vi "S7COMM - Timestamp to Siemens Date & Time.vi"(8 "error in":errorcluster, 11 "Time Stamp":timestamp) -> (0 "error out":errorcluster, 1 "DT":T1 {"Weekday" items=["Sunday"=1, "Monday"=2, "Tuesday"=3, "Wednesday"=4, "Thursday"=5, "Friday"=6, "Saturday"=7]; "Month" items=["Jan"=1, "Feb"=2, "Mar"=3, "Apr"=4, "May"=5, "Jun"=6, "Jul"=7, "Aug"=8, "Sep"=9, "Oct"=10, "Nov"=11, "Dec"=12]}, 3 "S7 DATE_AND_TIME":u8[](array[numeric]))   [LabVIEW 2014, in "S7NetCom.lvclass"]
uses:
  S7NetCom.lvclass
  S7COMM - Siemens Date & Time--cluster.ctl
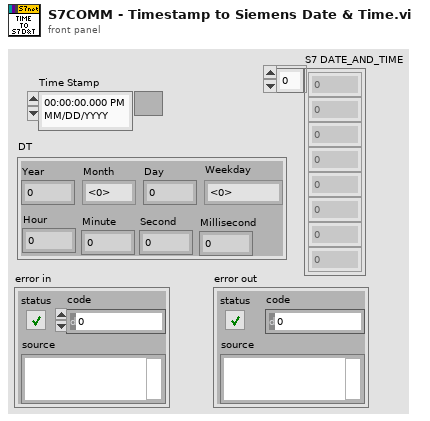
[diagram p1: front panel]
types:
  T1 = typedef "S7NetCom.lvclass/S7COMM - Siemens Date & Time--cluster.ctl" = cluster{"Year":i32, "Month":u8, "Day":u8, "Hour":u8, "Minute":u8, "Second":u8, "Millisecond":u32, "Weekday":u8}
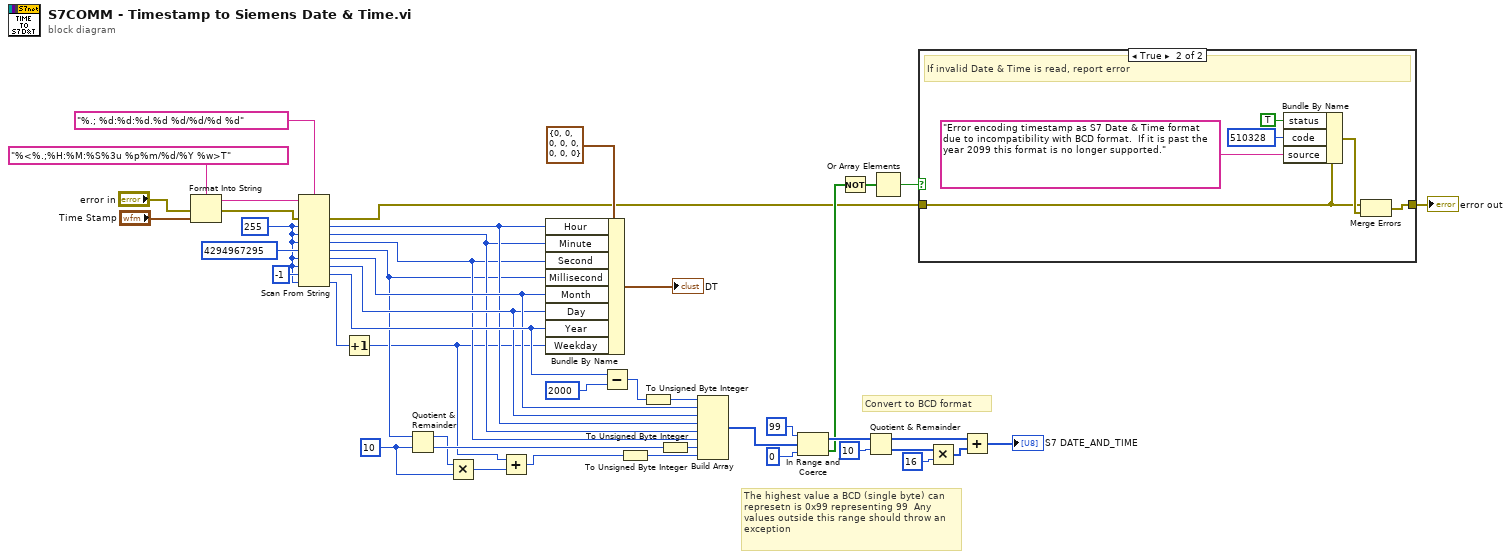
[diagram p0: block diagram]
diagram:
  w22 = u32 10 ("y")
  w36 = u8 255
  # "Convert to BCD format"
  # "The highest value a BCD (single byte) can represetn is 0x99 representing 99  Any values outside this range should throw an exception"
  n1 = Format Into String(format string="%<%.;%H:%M:%S%3u %p%m/%d/%Y %w>T", error in="error in", "Time Stamp") -> (resulting string=w44:string, error out=w39:errorcluster)  [unwired: 1 in]
  n2 = Scan From String(format string="%.; %d:%d:%d.%d %d/%d/%d %d", input string=w44, error in=w39, default 1=w36, default 2=w36, default 3=w36, default 4=u32 4294967295, default 5=w36, default 6=w36, default 7=-1 ("default value 7"), default 8=w36) -> (error out=w3:errorcluster, output 1=w28:u8, output 2=w27:u8, output 3=w26:u8, output 4=w25:u32, output 5=w30:u8, output 6=w29:u8, output 7=w34:i32, output 8=w35:u8)  [unwired: 1 in, 2 out]
  n3 = Increment(x=w35) -> (x+1=w20:u8)
  n4 = Quotient & Remainder(x=w25, y=w22) -> (x-y*floor(x/y)=w23:u32, floor(x/y)=w24:u32)
  n5 = Multiply(x=w23, y=w22) -> (x*y=w21:u32)
  n6 = Add(x=w20, y=w21) -> (x+y=w19:u32)
  n7 = Bundle By Name(cluster=T1 {"Year"=0, "Month"=0, "Day"=0, "Hour"=0, "Minute"=0, "Second"=0, "Millisecond"=0, "Weekday"=0} ("DT"), "Hour"=w28, "Minute"=w27, "Second"=w26, "Millisecond"=w25, "Month"=w30, "Day"=w29, "Year"=w34, "Weekday"=w20) -> (→"DT":T1)
  n8 = Subtract(x=w34, y=2000) -> (x-y=w32:i32)
  n9 = To Unsigned Byte Integer(number=w19) -> (unsigned 8bit integer=w17:u8)
  n10 = To Unsigned Byte Integer(number=w32) -> (unsigned 8bit integer=w31:u8)
  n11 = To Unsigned Byte Integer(number=w24) -> (unsigned 8bit integer=w18:u8)
  n12 = Build Array(w31, w30, w29, w28, w27, w26, w18, w17) -> (w16:u8[])
  n13 = In Range and Coerce(upper limit=u8 99, x=w16, lower limit=u8 0) -> (coerced(x)=w12:u8[], In Range?=w11:bool[])
  n14 = Not(x=w11) -> (.not. x?=w15:bool[])
  n15 = Quotient & Remainder(x=w12, y=u8 10) -> (x-y*floor(x/y)=w5:u8[], floor(x/y)=w6:u8[])
  n16 = Or Array Elements(Boolean array=w15) -> (logical OR=w2:bool)
  n17 = case shown="True" w2 {
    tunnel: w3 -> [w46 w47]
    tunnel: [w46 w52] -> w1
    frame False {
    }
    frame True {
      # "If invalid Date & Time is read, report error"
      n18 = Bundle By Name(cluster=w47, "status"=TRUE, "code"=510328, "source"="Error encoding timestamp as S7 Date & Time format due to incompatibility with BCD format.  If it is past the year 2099 this format is no longer supported.") -> (w48:errorcluster)
      n19 = Merge Errors(w47, w48) -> (w52:errorcluster)
    }
  }
  "error out" <- w1
  n20 = Multiply(x=w6, y=u8 16) -> (x*y=w8:u8[])
  n21 = Add(x=w5, y=w8) -> (x+y=→"S7 DATE_AND_TIME":u8[])
